vi "List Zip File Contents.vi"(8 "error in (no error)":errorcluster, 11 "Package File Path":path) -> (0 "error out":errorcluster, 1 "file infos":T1[](array[typedef]) {"file timestamp" format="%<%H:%M:%S\n%d/%m/%Y>T"; "external fa" format="%.0x"; "internal fa" format="%.0x"; "crc" format="%.0x"}, 2 "file names":string[](array[string]), 3 "dup Package File Path":path, 4 "global comment":string)   [LabVIEW 2019, in "Command-Line Zip.lvlib"]
doc: "Lists all the information contained in the file of an unzip session."
uses:
  <userlib>/_OpenG.lib/lvzip/lvzip.llb/ZLIB File Info__ogtk.ctl
  Command-Line Zip.lvlib
panel:
  out "standard output 2":string
  out "standard output":string
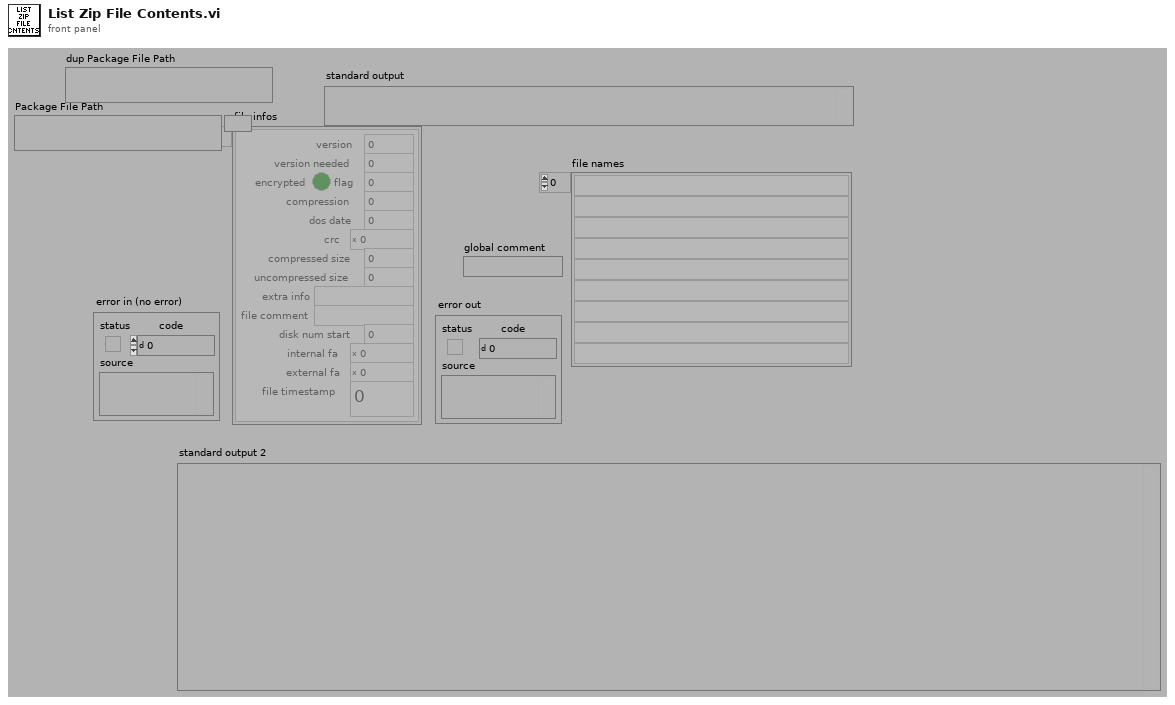
[diagram p1: front panel]
types:
  T1 = typedef "ZLIB File Info__ogtk.ctl" = cluster{"version":u32, "version needed":u32, "encrypted":bool, "flag":u32, "compression":i32, "dos date":u32, "crc":u32, "compressed size":u32, "uncompressed size":u32, "extra info":string, "file comment":string, "disk num start":u32, "internal fa":u32, "external fa":u32, "file timestamp":u32}
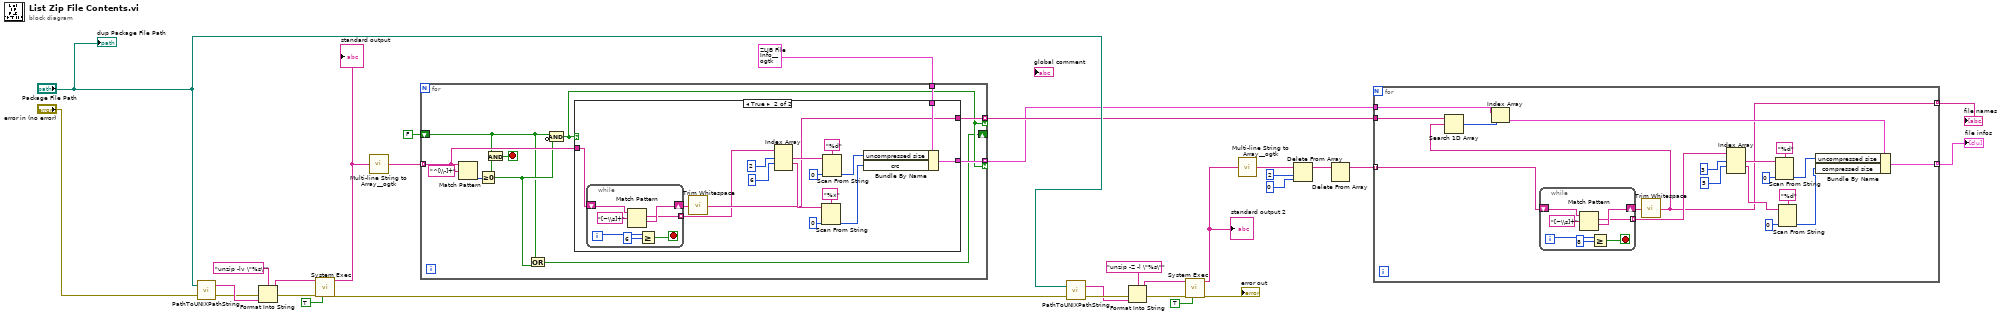
[diagram p0: block diagram]
diagram:
  n1 = call <vilib>:"PathToUNIXPathString.vi"("error in (no error)"="error in (no error)", "LV Path"="Package File Path") -> ("error out"=w25:errorcluster, "UNIX Path"=w26:string)
  n2 = Format Into String(format string="unzip -lv \"%s\"" ("command line"), error in=w25, w26) -> (resulting string=w29:string, error out=w28:errorcluster)  [unwired: 1 in]
  n3 = call <vilib>:"System Exec.vi"("run minimized? (F)"=TRUE, "error in (no error)"=w28, "command line"=w29) -> ("error out"=w13:errorcluster, "standard output"=w23:string)  [unwired: 5 in, 2 out]
  "standard output" <- w23
  n4 = call <userlib>:"Multi-line String to Array__ogtk.vi"("string"=w23) -> ("lines"=w22:string[])
  n5 = for {
    tunnel: w22 -> [w38] mode=indexing
    shift-right: [w31] -> _
    shift-left: FALSE -> [w32]
    tunnel: T1 {"version"=0, "version needed"=0, "encrypted"=FALSE, "flag"=0, "compression"=0, "dos date"=0, "crc"=0, "compressed size"=0, "uncompressed size"=0, "extra info"="", "file comment"="", "disk num start"=0, "internal fa"=0, "external fa"=0, "file timestamp"=0} ("file info") -> [w37]
    tunnel: [w36] -> w4 mode=indexing if=w34
    tunnel: [w35] -> w3 mode=indexing if=w34
    stop <- w39 stop-if-true
    n6 = Match Pattern(string=w38, regular expression="^[\\-]+") -> (offset past match=w40:i32)  [unwired: 1 in, 3 out]
    n7 = Greater Or Equal To 0?(x=w40) -> (x >= 0?=w33:bool)
    n8 = And(x=w32, y=w33) -> (x .and. y?=w39:bool)
    n9 = Or(x=w32, y=w33) -> (x .or. y?=w31:bool)
    n10 = Compound Arithmetic op=AND(w32, invert w33) -> (w34:bool)
    n11 = case shown="True" w34 {
      tunnel: w38 -> [_ w45]
      tunnel: w37 -> [_ w53]
      tunnel: [_ w43] -> w36
      tunnel: [_ w51] -> w35
      frame False {
      }
      frame True {
        n12 = while {
          shift-right: [w62] -> w44
          shift-left: w45 -> [w64]
          tunnel: [w61] -> w42 mode=indexing
          i -> [w60]
          stop <- w58 stop-if-true
          n13 = Match Pattern(string=w64, regular expression="[~\\s]+") -> (match substring=w61:string, after substring=w62:string)  [unwired: 1 in, 2 out]
          n14 = Greater Or Equal?(x=w60, y=6) -> (x >= y?=w58:bool)
        }
        n15 = call <vilib>:"Trim Whitespace.vi"("string"=w44) -> ("trimmed string"=w43:string)  [unwired: 1 in]
        n16 = Index Array(array=w42, index #1=2 ("index"), index #2=6 ("index")) -> (element #1=w55:string, element #2=w47:string)  [unwired: 1 in, 1 out]
        n17 = Scan From String(format string="%x", input string=w47, default 1=u32 0 ("crc")) -> (output 1=w46:u32)  [unwired: 2 in, 3 out]
        n18 = Scan From String(format string="%d", input string=w55, default 1=u32 0 ("uncompressed size")) -> (output 1=w52:u32)  [unwired: 2 in, 3 out]
        n19 = Bundle By Name(cluster=w53, "uncompressed size"=w52, "crc"=w46) -> (w51:T1)
      }
    }
  }
  n20 = call <vilib>:"PathToUNIXPathString.vi"("error in (no error)"=w13, "LV Path"="Package File Path") -> ("error out"=w19:errorcluster, "UNIX Path"=w18:string)
  n21 = Format Into String(format string="unzip -Z -l \"%s\"" ("command line"), error in=w19, w18) -> (resulting string=w15:string, error out=w16:errorcluster)  [unwired: 1 in]
  n22 = call <vilib>:"System Exec.vi"("run minimized? (F)"=TRUE, "error in (no error)"=w16, "command line"=w15) -> ("error out"=→"error out":errorcluster, "standard output"=w10:string)  [unwired: 5 in, 2 out]
  "standard output 2" <- w10
  n23 = call <userlib>:"Multi-line String to Array__ogtk.vi"("string"=w10) -> ("lines"=w8:string[])
  n24 = Delete From Array(array=w8, length=2, index=0) -> (array with subset deleted=w7:string[])  [unwired: 1 out]
  n25 = Delete From Array(array=w7) -> (array with subset deleted=w6:string[])  [unwired: 2 in, 1 out]
  n26 = for {
    tunnel: w6 -> [w69] mode=indexing
    tunnel: [w65] -> w2 mode=indexing
    tunnel: [w83] -> w1 mode=indexing
    tunnel: w4 -> [w70]
    tunnel: w3 -> [w67]
    n27 = while {
      shift-right: [w88] -> w76
      shift-left: w69 -> [w90]
      tunnel: [w87] -> w75 mode=indexing
      i -> [w86]
      stop <- w84 stop-if-true
      n28 = Match Pattern(string=w90, regular expression="[~\\s]+") -> (match substring=w87:string, after substring=w88:string)  [unwired: 1 in, 2 out]
      n29 = Greater Or Equal?(x=w86, y=8) -> (x >= y?=w84:bool)
    }
    n30 = call <vilib>:"Trim Whitespace.vi"("string"=w76) -> ("trimmed string"=w65:string)  [unwired: 1 in]
    n31 = Search 1D Array(1D array=w70, element=w65) -> (index of element=w68:i32)  [unwired: 1 in]
    n32 = Index Array(array=w67, index=w68) -> (element=w66:T1)
    n33 = Index Array(array=w75, index #1=3 ("index"), index #2=5 ("index")) -> (element #1=w80:string, element #2=w72:string)  [unwired: 1 in, 1 out]
    n34 = Scan From String(format string="%d", input string=w80, default 1=u32 0 ("uncompressed size")) -> (output 1=w78:u32)  [unwired: 2 in, 3 out]
    n35 = Scan From String(format string="%d", input string=w72, default 1=u32 0 ("uncompressed size")) -> (output 1=w71:u32)  [unwired: 2 in, 3 out]
    n36 = Bundle By Name(cluster=w66, "uncompressed size"=w78, "compressed size"=w71) -> (w83:T1)
  }
  "file names" <- w2
  "file infos" <- w1
  "dup Package File Path" <- "Package File Path"
